vi "cam0-输出颗粒信息.vi"(5 "截图左上Y":dbl, 7 "截图左上X":dbl, 9 "白条面积限度":dbl=200.0 format="%#_13g", 10 "颗粒分析结果":dbl[][](array[numeric]) format="%.2f") -> (0 "白条ok":bool, 1 "最大颗粒面积":dbl, 2 "矩形框":T1)   [LabVIEW 2018]
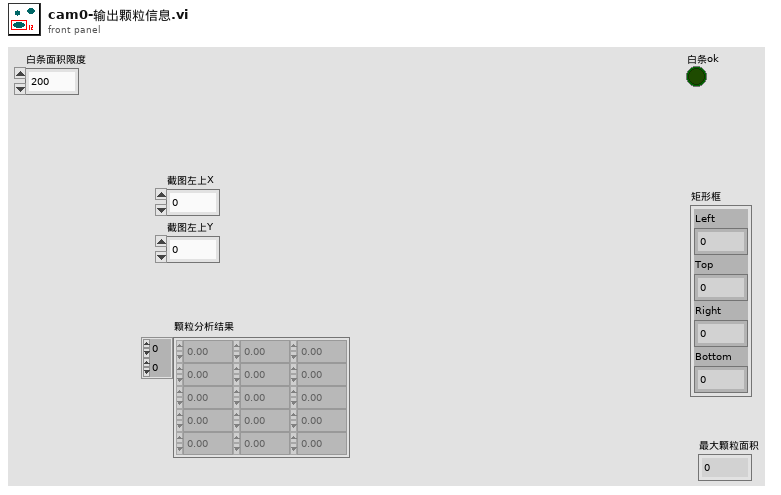
[diagram p1: front panel]
types:
  T1 = cluster{"Left":i32, "Top":i32, "Right":i32, "Bottom":i32}
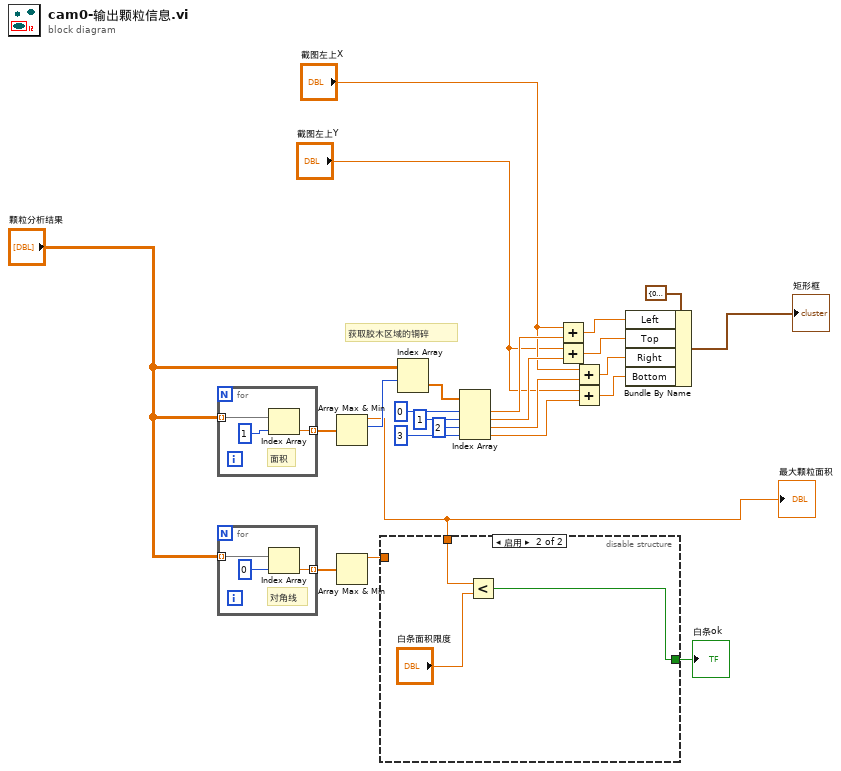
[diagram p0: block diagram]
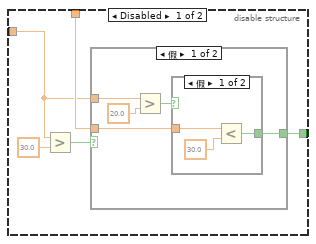
[diagram p2: hidden frame]
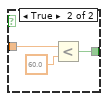
[diagram p3: hidden frame]
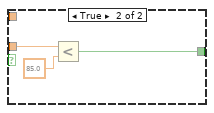
[diagram p4: hidden frame]
diagram:
  # "获取胶木区域的铜碎"
  n1 = for {
    tunnel: "颗粒分析结果" -> [w27] mode=indexing
    tunnel: [w26] -> w9 mode=indexing
    # "面积"
    n2 = Index Array(array=w27, index=1 ("索引")) -> (element=w26:dbl)
  }
  n3 = for {
    tunnel: "颗粒分析结果" -> [w30] mode=indexing
    tunnel: [w29] -> w5 mode=indexing
    # "对角线"
    n4 = Index Array(array=w30, index=0 ("索引")) -> (element=w29:dbl)
  }
  n5 = Array Max & Min(array=w9) -> (max value=w3:dbl, max index (indices)=w24:i32)  [unwired: 2 out]
  "最大颗粒面积" <- w3
  n6 = Array Max & Min(array=w5) -> (max value=w1:dbl)  [unwired: 3 out]
  n7 = disable-structure shown="启用" {
    disable-tunnel: w3 -> [w35 w52]
    disable-tunnel: [w34 w50] -> w2
    disable-tunnel: w1 -> [w31 _]
    frame Disabled {
      n8 = Greater?(x=w31, y=30.0) -> (0:w32:bool)
      n9 = case shown="假" w32 {
        tunnel: w35 -> [w37 w48]
        tunnel: [w36 w47] -> w34
        tunnel: w31 -> [w38 _]
        frame False {
          n10 = Greater?(x=w38, y=20.0) -> (0:w39:bool)
          n11 = case shown="假" w39 {
            tunnel: w37 -> [w43 w46]
            tunnel: [w41 w44] -> w36
            frame False {
              n12 = Less?(x=w43, y=30.0) -> (x < y?=w41:bool)
            }
            frame True {
              n13 = Less?(x=w46, y=60.0) -> (x < y?=w44:bool)
            }
          }
        }
        frame True {
          n14 = Less?(x=w48, y=85.0) -> (x < y?=w47:bool)
        }
      }
    }
    frame Enabled {
      n15 = Less?(x=w52, y="白条面积限度") -> (x < y?=w50:bool)
    }
  }
  "白条ok" <- w2
  n16 = Index Array(array="颗粒分析结果", index (row)=w24) -> (element=w10:dbl[])  [unwired: 1 in]
  n17 = Index Array(array=w10, index #1=0 ("索引"), index #2=1 ("索引"), index #3=2 ("索引"), index #4=3 ("索引")) -> (element #1=w17:dbl, element #2=w16:dbl, element #3=w18:dbl, element #4=w19:dbl)
  n18 = Add(x="截图左上X", y=w17) -> (x+y=w23:dbl)
  n19 = Add(x="截图左上Y", y=w16) -> (x+y=w22:dbl)
  n20 = Add(x="截图左上X", y=w18) -> (x+y=w21:dbl)
  n21 = Add(x="截图左上Y", y=w19) -> (x+y=w20:dbl)
  n22 = Bundle By Name(cluster=T1 {"Left"=0, "Top"=0, "Right"=0, "Bottom"=0} ("Rectangle"), "Left"=w23, "Top"=w22, "Right"=w21, "Bottom"=w20) -> (→"矩形框":T1)
